vi "Plotter_Receive_Log_File_FGV.vi"() -> ()   [LabVIEW 2017]
uses:
  <vilib>/Utility/file.llb/Write Delimited Spreadsheet (string).vi
panel:
  in  "Initialize ?":bool
  out "error out":errorcluster
  in  "error in (no error)":errorcluster
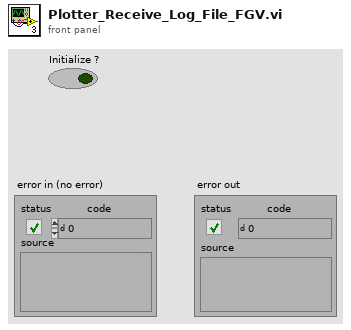
[diagram p1: front panel]
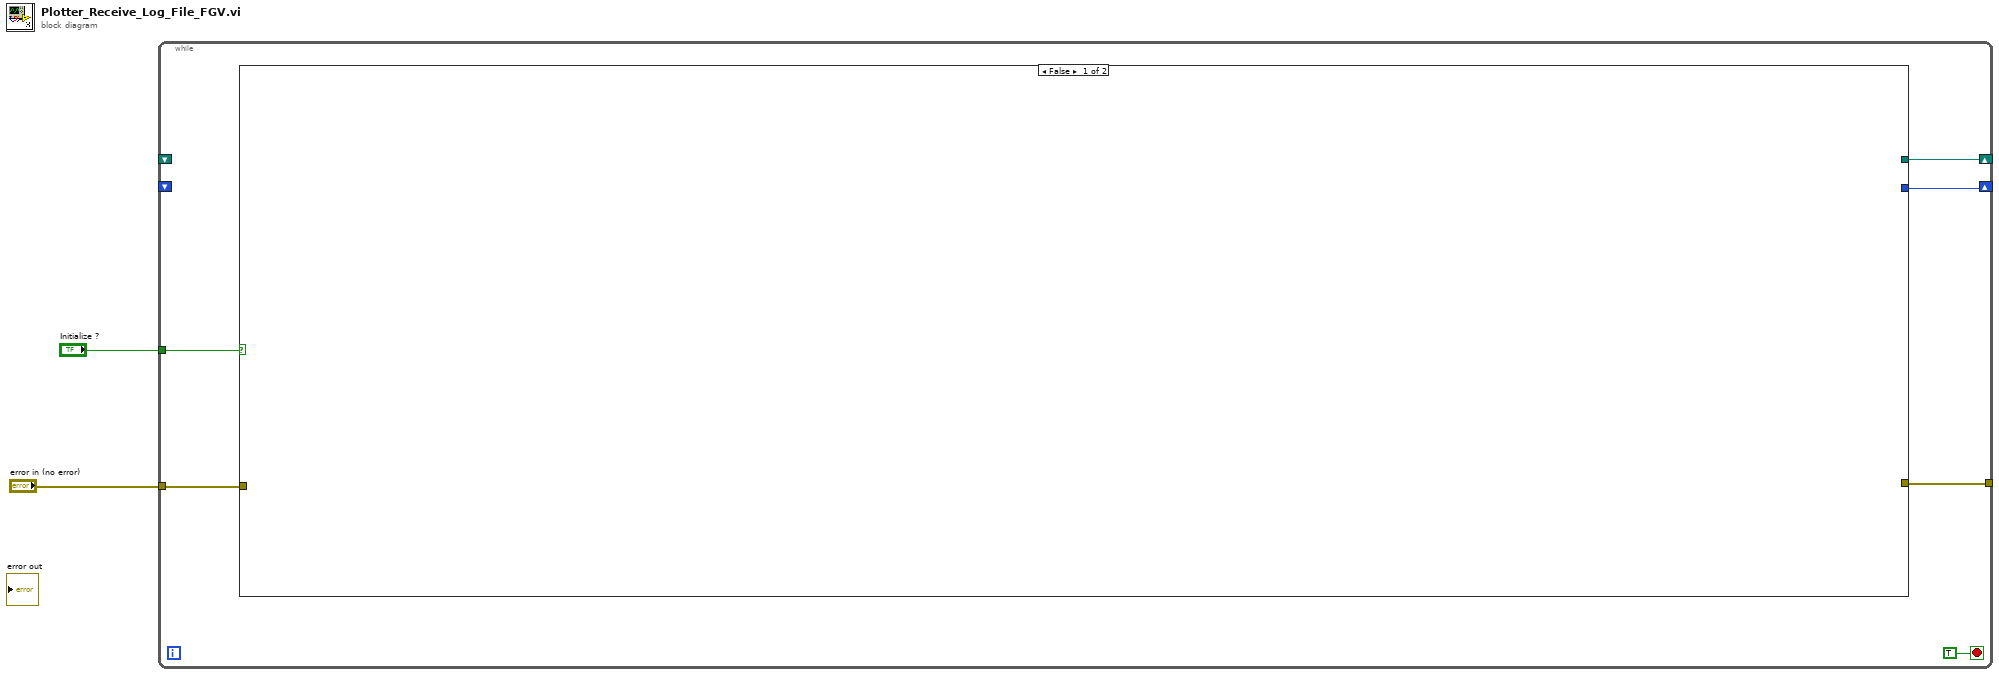
[diagram p0: block diagram]
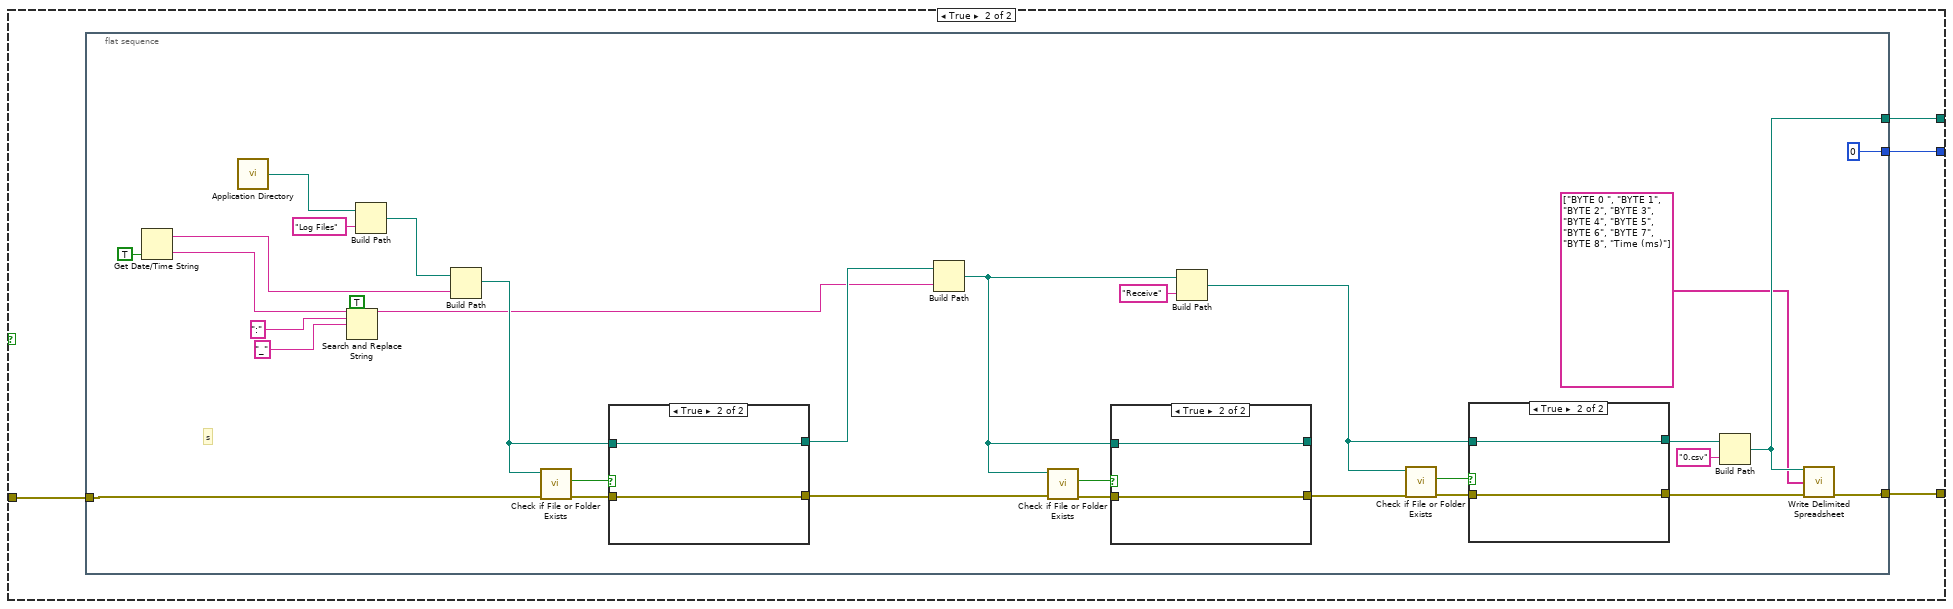
[diagram p2: hidden frame]
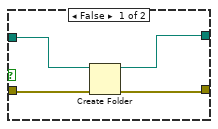
[diagram p3: hidden frame]
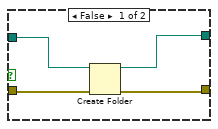
[diagram p4: hidden frame]
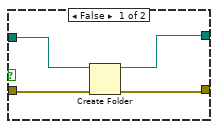
[diagram p5: hidden frame]
diagram:
  n1 = while {
    tunnel: "error in (no error)" -> [w8]
    tunnel: "Initialize ?" -> [w7]
    tunnel: [w5] -> _
    shift-right: [w4] -> _
    shift-left: _ -> [_]
    shift-right: [w3] -> _
    shift-left: _ -> [_]
    stop <- TRUE stop-if-true
    n2 = case shown="False" w7 {
      tunnel: w8 -> [_ w12]
      tunnel: [_ w11] -> w5
      tunnel: [_ w10] -> w4
      tunnel: [_ w9] -> w3
      frame False {
      }
      frame True {
        n3 = flat-sequence {
          tunnel: w12 -> [w38]
          tunnel: [w14] -> w11
          tunnel: [w16] -> w10
          tunnel: [0] -> w9
          frame #0 {
            # "s"
            n4 = Get Date/Time String(want seconds? (F)=TRUE) -> (date string=w39:string, time string=w33:string)  [unwired: 2 in]
            n5 = call <vilib>:"Application Directory.vi"() -> ("Application Directory"=w42:path)
            n6 = Search and Replace String(replace all?=TRUE ("replace all? (F)"), input string=w33, search string=":", replace string="_" ("replace string (\"\")")) -> (result string=w29:string)  [unwired: 4 in, 3 out]
            n7 = Build Path(base path=w42, name or relative path="Log Files") -> (appended path=w40:path)
            n8 = Build Path(base path=w40, name or relative path=w39) -> (appended path=w35:path)
            n9 = call <vilib>:"Check if File or Folder Exists.vi"("error in (no error)"=w38, "path"=w35) -> ("error out"=w36:errorcluster, "file or folder exists?"=w37:bool)  [unwired: 7 in, 1 out]
            n10 = case shown="True" w37 {
              tunnel: w36 -> [w59 w61]
              tunnel: [w57 w61] -> w26
              tunnel: w35 -> [w58 w60]
              tunnel: [w56 w60] -> w34
              frame False {
                n11 = Create Folder(path (use dialog)=w58, error in=w59) -> (created path=w56:path, error out=w57:errorcluster)  [unwired: 1 in, 1 out]
              }
              frame True {
              }
            }
            n12 = Build Path(base path=w34, name or relative path=w29) -> (appended path=w25:path)
            n13 = call <vilib>:"Check if File or Folder Exists.vi"("error in (no error)"=w26, "path"=w25) -> ("error out"=w27:errorcluster, "file or folder exists?"=w28:bool)  [unwired: 7 in, 1 out]
            n14 = case shown="True" w28 {
              tunnel: w27 -> [w53 w55]
              tunnel: [w51 w55] -> w21
              tunnel: w25 -> [w52 w54]
              tunnel: [w50 w54] -> _
              frame False {
                n15 = Create Folder(path (use dialog)=w52, error in=w53) -> (created path=w50:path, error out=w51:errorcluster)  [unwired: 1 in, 1 out]
              }
              frame True {
              }
            }
            n16 = Build Path(base path=w25, name or relative path="Receive") -> (appended path=w20:path)
            n17 = call <vilib>:"Check if File or Folder Exists.vi"("error in (no error)"=w21, "path"=w20) -> ("error out"=w22:errorcluster, "file or folder exists?"=w23:bool)  [unwired: 7 in, 1 out]
            n18 = case shown="True" w23 {
              tunnel: w22 -> [w47 w49]
              tunnel: [w45 w49] -> w19
              tunnel: w20 -> [w46 w48]
              tunnel: [w44 w48] -> w18
              frame False {
                n19 = Create Folder(path (use dialog)=w46, error in=w47) -> (created path=w44:path, error out=w45:errorcluster)  [unwired: 1 in, 1 out]
              }
              frame True {
              }
            }
            n20 = Build Path(base path=w18, name or relative path="0.csv") -> (appended path=w16:path)
            n21 = call-poly <vilib>:"Write Delimited Spreadsheet.vi"("file path (dialog if empty)"=w16, "1D data"=string[] ["BYTE 0 ", "BYTE 1", "BYTE 2", "BYTE 3", "BYTE 4", "BYTE 5", "BYTE 6", "BYTE 7", "BYTE 8", "Time (ms)"], "error in (no error)"=w19) -> ("error out"=w14:errorcluster)  [unwired: 11 in, 1 out]
          }
        }
      }
    }
  }
